vi "FeatureLocation.vi"(8 "error in (no error)":errorcluster, 9 "Coordinate System":T3 {"Measurement System"."Axis Reference" items=["Direct", "Indirect"]; "Measurement System"."Angle (deg)" format="%.2f"; "Measurement System"."Origin"."Y" format="%.2f"; "Measurement System"."Origin"."X" format="%.2f"; "Reference System"."Axis Reference" items=["Direct", "Indirect"]; "Reference System"."Angle (deg)" format="%.2f"; "Reference System"."Origin"."Y" format="%.2f"; "Reference System"."Origin"."X" format="%.2f"}, 11 "Image":T2) -> (0 "error out":errorcluster, 1 "Vertical Edges":T4(array[cluster]) {"Point2 (Real-World)"."Y" format="%.2f"; "Point2 (Real-World)"."X" format="%.2f"; "Point1 (Real-World)"."Y" format="%.2f"; "Point1 (Real-World)"."X" format="%.2f"; "Point2 (Pixels)"."Y" format="%.2f"; "Point2 (Pixels)"."X" format="%.2f"; "Point1 (Pixels)"."Y" format="%.2f"; "Point1 (Pixels)"."X" format="%.2f"}, 2 "Horizontal Edges":T4(array[cluster]) {"Point2 (Real-World)"."Y" format="%.2f"; "Point2 (Real-World)"."X" format="%.2f"; "Point1 (Real-World)"."Y" format="%.2f"; "Point1 (Real-World)"."X" format="%.2f"; "Point2 (Pixels)"."Y" format="%.2f"; "Point2 (Pixels)"."X" format="%.2f"; "Point1 (Pixels)"."Y" format="%.2f"; "Point1 (Pixels)"."X" format="%.2f"}, 3 "Image 2":T2(plugin-control), 4 "Puck":T1(array[cluster]) {"Position"."Y" format="%.2f"; "Position"."X" format="%.2f"}, 5 "Players":T1(array[cluster]) {"Position"."Y" format="%.2f"; "Position"."X" format="%.2f"})   [LabVIEW 2017]
uses:
  <vilib>/vision/Image Controls.llb/IMAQ Image.ctl
panel:
  out "Number of Pucks Found":i32
  out "Number of Players Found":i32
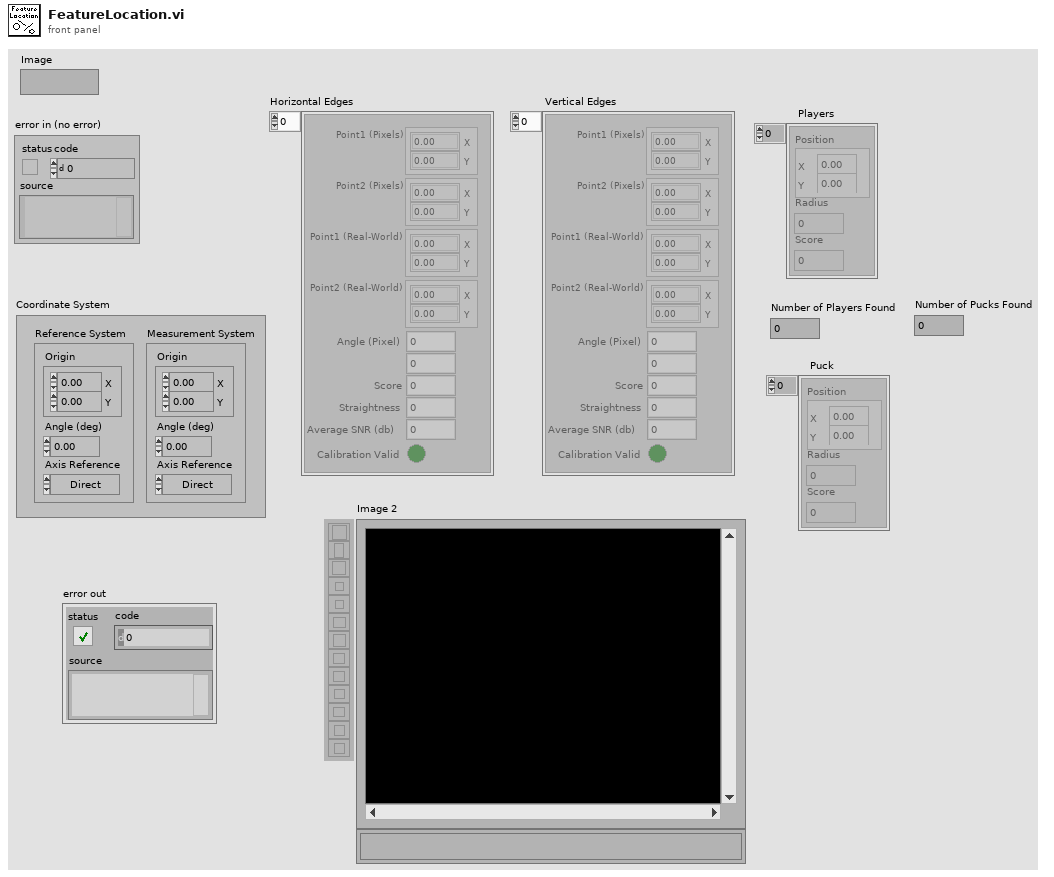
[diagram p1: front panel]
types:
  T1 = cluster{"Position":cluster{"X":sgl, "Y":sgl}, "Radius":dbl, "Score":dbl}[]
  T2 = typedef "IMAQ Image.ctl" = refnum<image>
  T3 = typedef "IMAQ Coordinate System" = cluster{"Reference System":cluster{"Origin":cluster{"X":sgl, "Y":sgl}, "Angle (deg)":sgl, "Axis Reference":u32}, "Measurement System":cluster{"Origin":cluster{"X":sgl, "Y":sgl}, "Angle (deg)":sgl, "Axis Reference":u32}}
  T4 = cluster{"Point1 (Pixels)":cluster{"X":sgl, "Y":sgl}, "Point2 (Pixels)":cluster{"X":sgl, "Y":sgl}, "Point1 (Real-World)":cluster{"X":sgl, "Y":sgl}, "Point2 (Real-World)":cluster{"X":sgl, "Y":sgl}, "Angle (Pixel)":dbl, "Angle (Real-World)":dbl, "Score":dbl, "Straightness":dbl, "Average SNR (db)":dbl, "Calibration Valid":bool}[]
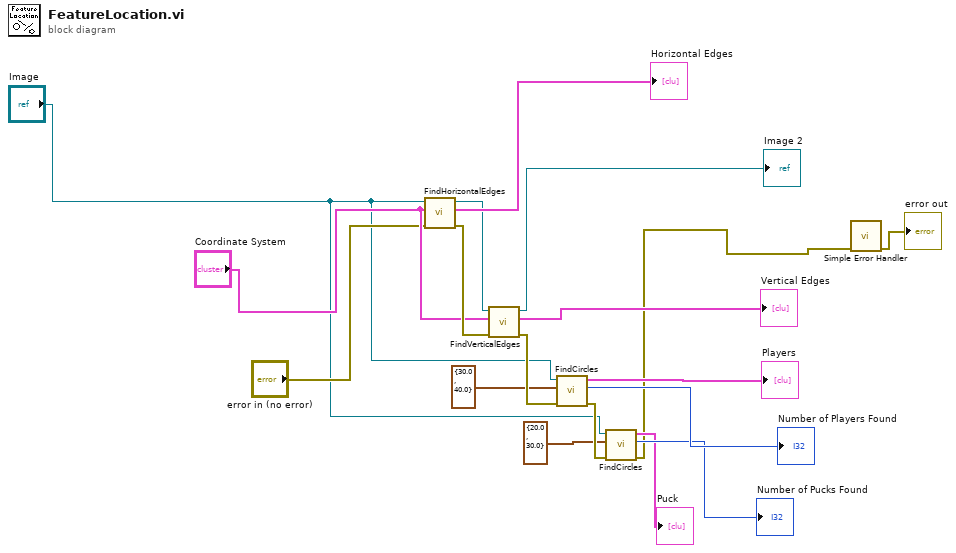
[diagram p0: block diagram]
diagram:
  n1 = call "FindHorizontalEdges.vi"("error in (no error)"="error in (no error)", "Coordinate System"="Coordinate System", "Image"="Image") -> ("error out"=w16:errorcluster, "Straight Edges"=→"Horizontal Edges":T4, "Image 2"=w14:T2)  [unwired: 6 in]
  n2 = call "FindVerticalEdges.vi"("error in (no error)"=w16, "Coordinate System"="Coordinate System", "Image"=w14) -> ("error out"=w12:errorcluster, "Straight Edges"=→"Vertical Edges":T4, "Image 2"=→"Image 2":T2)  [unwired: 6 in]
  n3 = call "FindCircles.vi"("error in (no error)"=w12, "Circle Descriptor"=cluster{"Min Radius":dbl, "Max Radius":dbl} {"Min Radius"=30.0, "Max Radius"=40.0}, "Image"="Image") -> ("error out"=w7:errorcluster, "Number of Matches Returned"=→"Number of Players Found":i32, "Circles"=→"Players":T1)  [unwired: 6 in]
  n4 = call "FindCircles.vi"("error in (no error)"=w7, "Circle Descriptor"=cluster{"Min Radius":dbl, "Max Radius":dbl} {"Min Radius"=20.0, "Max Radius"=30.0}, "Image"="Image") -> ("error out"=w3:errorcluster, "Number of Matches Returned"=→"Number of Pucks Found":i32, "Circles"=→"Puck":T1)  [unwired: 6 in]
  n5 = call <vilib>:"Simple Error Handler.vi"("error in (no error)"=w3) -> ("error out"=→"error out":errorcluster)  [unwired: 4 in, 4 out]
